vi "M Water Cells.vi"(11 "EV3 in":T1) -> ()   [LabVIEW 2016]
uses:
  <vilib>/NXT/Subs/LVHSConnector.ctl
  <vilib>/NXT/LegoClasses/BrickReference/BrickReference.lvclass
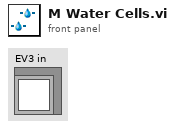
[diagram p1: front panel]
types:
  T1 = typedef "LVHSConnector.ctl" = refnum<class "BrickReference.lvclass">
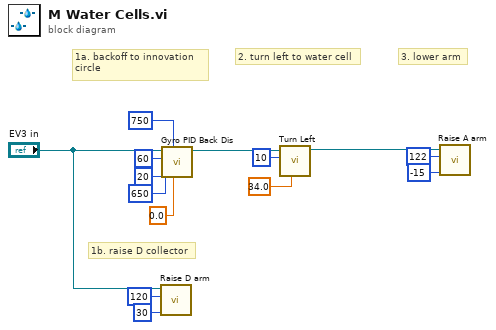
[diagram p0: block diagram]
diagram:
  # "3. lower arm"
  # "2. turn left to water cell"
  # "1b. raise D collector"
  # "1a. backoff to innovation\ncircle"
  n1 = call "Raise D arm.vi"("Power"=i8 30, "Rotation"=120, "EV3 in"="EV3 in") -> ()  [unwired: 8 in, 1 out]
  n2 = call "Gyro PID Back Dis.vi"("Target angle"=sgl 0.0, "Threshold to stop"=750, "Threshold to slow"=650, "Min. speed"=20, "Max. speed"=60, "EV3 in"="EV3 in") -> ("EV3 out"=w7:T1)  [unwired: 5 in]
  n3 = call "Turn Left.vi"("Turning angle"=sgl 34.0, "Motor B (right)"=i8 10, "EV3 in"=w7) -> ("EV3 out"=w4:T1)  [unwired: 8 in]
  n4 = call "Raise A arm.vi"("Power"=i8 -15, "Rotation"=122, "EV3 in"=w4) -> ()  [unwired: 8 in, 1 out]
